vi "Unlock Publication.vi"(6 "Publisher ID":string, 8 "error in (no error)":errorcluster, 9 "Datum Type":variant, 10 "Datum Name":string, 11 "IMediator In":refnum<class "IMediator.lvclass">) -> (0 "error out":errorcluster, 3 "IMediator Out":refnum<class "IMediator.lvclass">)   [LabVIEW 2015, in "IMediator.lvlib" / "IMediator.lvclass"]
doc: "<License>\nCopyright © 2017 Composed Systems, LLC | All rights reserved\nwww.composed.io\n\nAuthor: Ethan Stern <ethan.stern@composed.io>\n\nThis software is provided \"AS IS\" WITHOUT WARRANTIES, either express or implied, AND IS FOR EDUCATIONAL PURPOSES ONLY.\n</License>"
uses:
  IMediator.lvclass
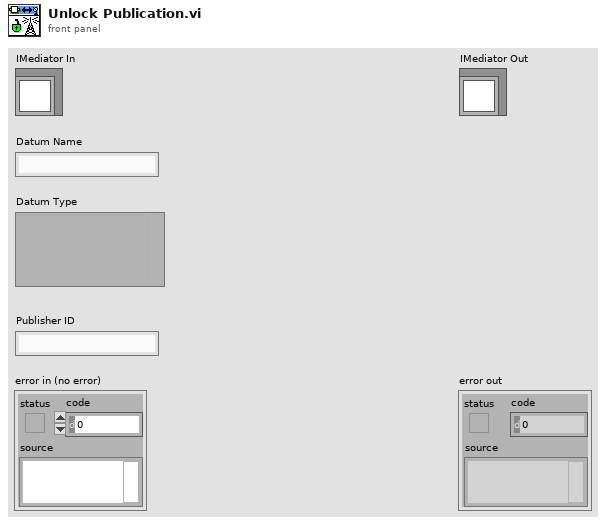
[diagram p1: front panel]
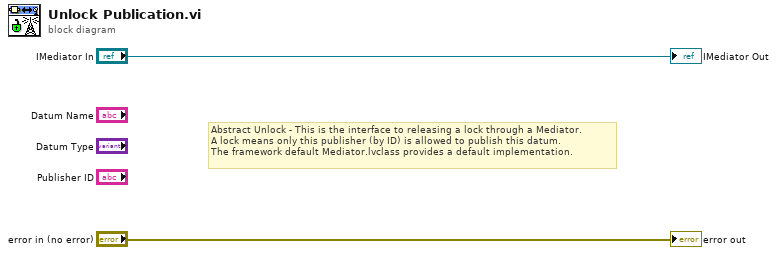
[diagram p0: block diagram]
diagram:
  # "Abstract Unlock - This is the interface to releasing a lock through a Mediator.\nA lock means only this publisher (by ID) is allowed to publish this datum.\nThe framework default Mediator.lvclass provides a default implementation."
  "error out" <- "error in (no error)"
  "IMediator Out" <- "IMediator In"
